vi "REM IO - Get Slave Data.vi"(8 "error in (no error)":errorcluster caption="Fehler (Eingang, kein Fehler)", 11 "EtherCAT Slave In":T9 {"VS ref" format="%.0x"}) -> (0 "error out":errorcluster caption="Fehler (Ausgang)", 3 "EtherCAT Slave out":T1 {"I/O Output Data"."BD Refs"."Data Reference" format="%.0x"; "I/O Input Data"."BD Refs"."Data Reference" format="%.0x"; "I/O Output Vars"."VS ref" format="%.0x"; "I/O Imput Vars"."VS ref" format="%.0x"; "VS ref" format="%.0x"})   [LabVIEW 2015, in "Scan Engine Custom Device.lvlib"]
uses:
  Scan Engine Custom Device.lvlib
  <vilib>/NI Veristand/Custom Device API/Custom Device Item Ref.ctl
  Type Defs/Generic ECAT Slave Data Cluster.ctl
  Type Defs/Generic ECAT Slave IOV Cluster.ctl
  Type Defs/UDV Data Type.ctl
  Type Defs/Input Data.ctl
  <vilib>/NI Veristand/Custom Device API/Block Data Reference.ctl
  <vilib>/NI Veristand/Custom Device API/Data Reference.ctl
  Type Defs/Output Data.ctl
  Globals/Property Strings.vi
  <vilib>/NI Veristand/Custom Device API/Custom Device API.lvlib
  <resource>/objmgr/IndComECAT.rc
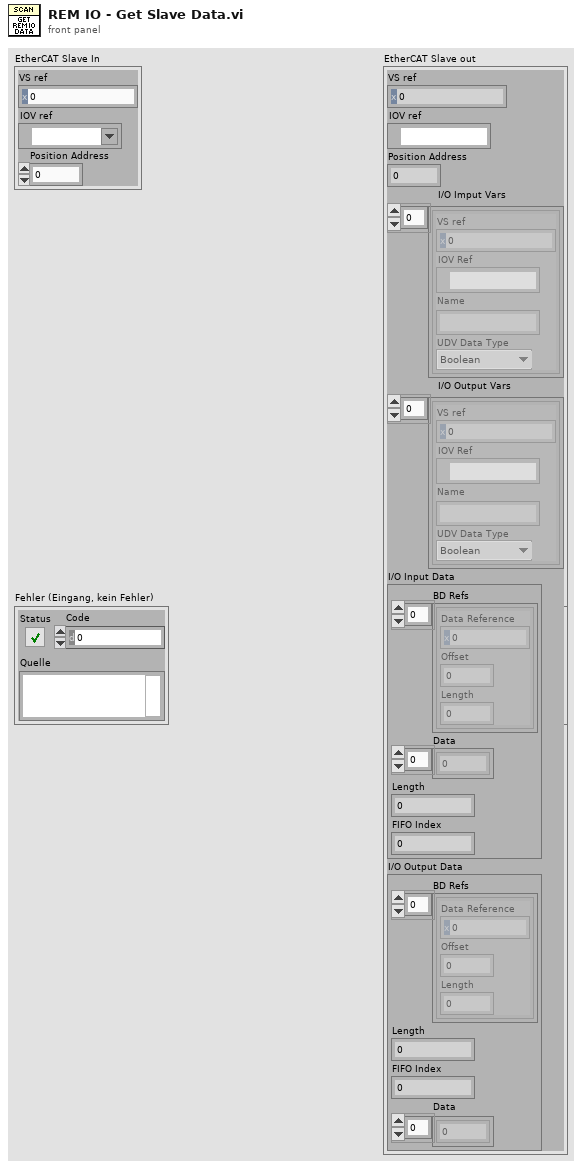
[diagram p1: front panel]
types:
  T1 = typedef "Scan Engine Custom Device.lvlib/Generic ECAT Slave Data Cluster.ctl" = cluster{"VS ref":T2, "IOV ref":refnum<k21>, "Position Address":u16, "I/O Imput Vars ":T3[], "I/O Output Vars":T3[], "I/O Input Data":T5, "I/O Output Data":T8}
  T2 = typedef "Custom Device API.lvlib/Custom Device Item Ref.ctl" = u64
  T3 = typedef "Scan Engine Custom Device.lvlib/Generic ECAT Slave IOV Cluster.ctl" = cluster{"VS ref":T2, "IOV Ref":refnum<k21>, "Name":string, "UDV Data Type":T4}
  T4 = typedef "Scan Engine Custom Device.lvlib/UDV Data Type.ctl" = enum16{"Boolean", "Fixed Point", "Int8", "Int16", "Int32", "Int64", "U32 Bit Field", "UInt8", "UInt16", "UInt32", "UInt64", "Other"}
  T5 = typedef "Scan Engine Custom Device.lvlib/Input Data.ctl" = cluster{"BD Refs":T6[], "Data":dbl[], "Length":i32, "FIFO Index":i32}
  T6 = typedef "Custom Device API.lvlib/Block Data Reference.ctl" = cluster{"Data Reference":T7, "Offset":u64, "Length":u64}
  T7 = typedef "Custom Device API.lvlib/Data Reference.ctl" = i32
  T8 = typedef "Scan Engine Custom Device.lvlib/Output Data.ctl" = cluster{"BD Refs":T6[], "Length":i32, "FIFO Index":i32, "Data":dbl[]}
  T9 = cluster{"VS ref":T2, "IOV ref":refnum<k21>, "Position Address":u16}
  T10 = cluster{"Input VS Refs":T2[], "Output VS Refs":T2[]}
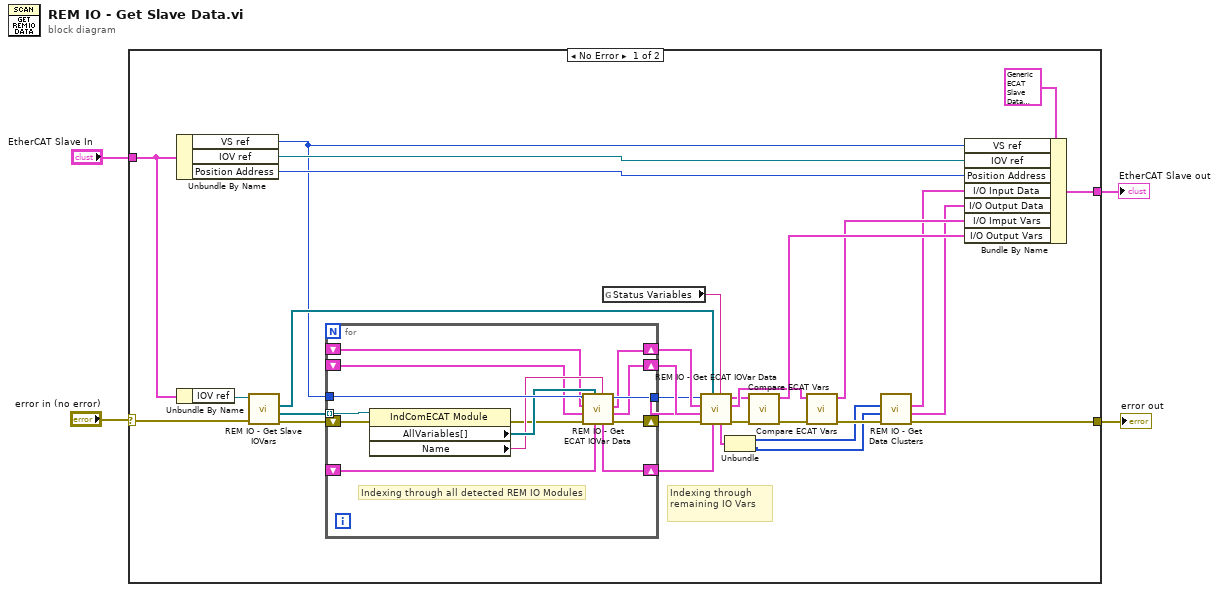
[diagram p0: block diagram]
diagram:
  n1 = case shown="No Error" "error in (no error)" {
    selector: "error in (no error)" -> [w29 w49]
    tunnel: "EtherCAT Slave In" -> [w34 _]
    tunnel: [w15 w49] -> w3
    tunnel: [w5 _] -> w2
    frame No Error {
      # "Indexing through remaining IO Vars"
      n2 = Unbundle By Name(w34) -> ("VS ref"=w8:T2, "IOV ref"=w32:refnum<k21>, "Position Address"=w33:u16)
      n3 = Unbundle By Name(w34) -> ("IOV ref"=w28:refnum<k21>)
      n4 = call "REM IO - Get Slave IOVars.vi"("error in (no error)"=w29, "ECAT Slave in"=w28) -> ("error IO"=w12:errorcluster, "REM IO Modules"=w14:refnum<k21>[], "ECAT Variablenobjekt"=w13:refnum<k21>[])  [unwired: 6 in, 1 out]
      n5 = for {
        shift-right: [w40] -> w21
        shift-left: w12 -> [w48]
        tunnel: w14 -> [w47] mode=indexing
        tunnel: w8 -> [w46]
        tunnel: [w43] -> w20
        shift-right: [w42] -> w23
        shift-left: _ -> [w37]
        shift-right: [w41] -> w22
        shift-left: _ -> [w36]
        shift-right: [w38] -> w7
        shift-left: _ -> [w35]
        # "Indexing through all detected REM IO Modules"
        n6 = property class="IndComECAT Module"(reference=w47, error in=w48) -> (error out=w39:errorcluster, "AllVariables[]"=w45:refnum<k21>[], "Name"=w44:string)  [unwired: 1 out]
        n7 = call "REM IO - Get ECAT IOVar Data.vi"("Section Name"=w44, "VS Refs In"=w35, "ECAT Variablenobjekt"=w45, "Fehler (Eingang, kein Fehler)"=w39, "I/O Output Vars In"=w36, "I/O Imput Vars In"=w37, "VS ref"=w46) -> ("Fehler (Ausgang)"=w40:errorcluster, "I/O Output Vars Out"=w41:T3[], "I/O Imput Vars Out"=w42:T3[], "VS ref 2"=w43:T2, "VS Refs Out"=w38:T10)
      }
      n8 = global read "Property Strings.vi" "Status Variables"() -> (w16:string)
      n9 = call "REM IO - Get ECAT IOVar Data.vi"("Section Name"=w16, "VS Refs In"=w7, "ECAT Variablenobjekt"=w13, "Fehler (Eingang, kein Fehler)"=w21, "I/O Output Vars In"=w22, "I/O Imput Vars In"=w23, "VS ref"=w20) -> ("Fehler (Ausgang)"=w11:errorcluster, "I/O Output Vars Out"=w9:T3[], "I/O Imput Vars Out"=w10:T3[], "VS Refs Out"=w19:T10)  [unwired: 1 out]
      n10 = Unbundle(w19) -> ("Input VS Refs"=w18:T2[], "Output VS Refs"=w17:T2[])
      n11 = call "Compare ECAT Vars.vi"("Fehler (Eingang, kein Fehler)"=w11, "I/O Output Vars (Eingang)"=w9) -> ("Fehler (Ausgang)"=w31:errorcluster, "I/O Output Vars (Ausgang)"=w27:T3[])  [unwired: 8 in]
      n12 = call "Compare ECAT Vars.vi"("Fehler (Eingang, kein Fehler)"=w31, "I/O Output Vars (Eingang)"=w10) -> ("Fehler (Ausgang)"=w30:errorcluster, "I/O Output Vars (Ausgang)"=w26:T3[])  [unwired: 8 in]
      n13 = call "REM IO - Get Data Clusters.vi"("error in (no error)"=w30, "Output VS Refs"=w17, "Input VS Refs"=w18) -> ("error out"=w15:errorcluster, "I/O Output Data"=w24:T8, "I/O Input Data"=w25:T5)  [unwired: 6 in]
      n14 = Bundle By Name(cluster=T1 {"VS ref"=0, "IOV ref"="", "Position Address"=0, "I/O Imput Vars "=[], "I/O Output Vars"=[], "I/O Input Data"={"BD Refs"=[], "Data"=[], "Length"=0, "FIFO Index"=0}, "I/O Output Data"={"BD Refs"=[], "Length"=0, "FIFO Index"=0, "Data"=[]}} ("EtherCAT Slave"), "VS ref"=w8, "IOV ref"=w32, "Position Address"=w33, "I/O Input Data"=w25, "I/O Output Data"=w24, "I/O Imput Vars"=w26, "I/O Output Vars"=w27) -> (w5:T1)
    }
    frame Error {
    }
  }
  "error out" <- w3
  "EtherCAT Slave out" <- w2
